vi "Read Slider Props.vi"(8 "error in (no error)":errorcluster, 11 "Slider in":refnum<vi>) -> (0 "error out":errorcluster, 2 "Slider Props":T1, 3 "Slider":refnum<vi>)   [LabVIEW 2020, in "VolatusGUIEditorCore.lvlib"]
uses:
  VolatusGUIEditorCore.lvlib
  Slider Props.ctl
  Fill Style.ctl
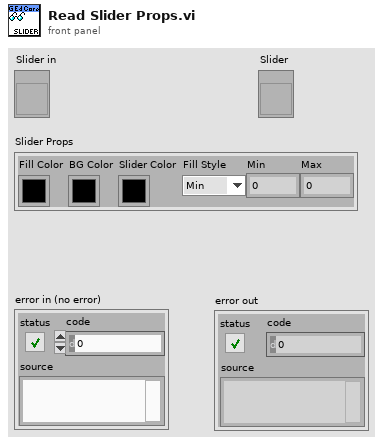
[diagram p1: front panel]
types:
  T1 = typedef "VolatusGUIEditorCore.lvlib/Slider Props.ctl" = cluster{"Fill Color":u32, "BG Color":u32, "Slider Color":u32, "Fill Style":T2, "Min":dbl, "Max":dbl}
  T2 = typedef "VolatusGUIEditorCore.lvlib/Fill Style.ctl" = enum16{"Min", "Max", "None"}
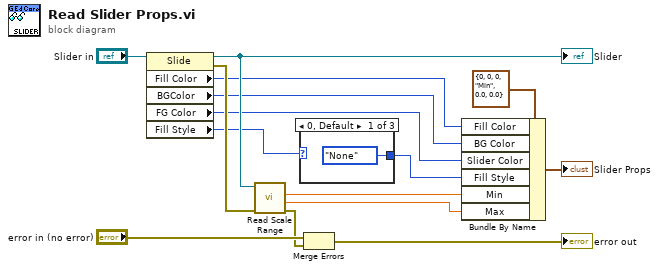
[diagram p0: block diagram]
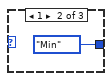
[diagram p2: hidden frame]
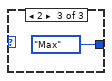
[diagram p3: hidden frame]
diagram:
  n1 = property class="Slide"(reference="Slider in") -> (reference out=w13:refnum<vi>, error out=w15:errorcluster, "Fill Color"=w10:u32, "BGColor"=w9:u32, "FG Color"=w8:u32, "Fill Style"=w5:i32)  [unwired: 1 in]
  "Slider" <- w13
  n2 = call "Read Scale Range.vi"("error in (no error)"=w15, "Ctl Refnum in"=w13) -> ("error out"=w3:errorcluster, "Max"=w6:dbl, "Min"=w7:dbl)  [unwired: 6 in, 1 out]
  n3 = case shown="0, Default" w5 {
    tunnel: [Fill_Style."None" ("Fill Style") Fill_Style."Min" ("Fill Style") Fill_Style."Max" ("Fill Style")] -> w1
    frame 0, Default {
    }
    frame 1 {
    }
    frame 2 {
    }
  }
  n4 = Merge Errors("error in (no error)", w3) -> (→"error out":errorcluster)
  n5 = Bundle By Name(cluster=T1 {"Fill Color"=0, "BG Color"=0, "Slider Color"=0, "Fill Style"=enum."Min", "Min"=0.0, "Max"=0.0} ("Slider Props"), "Fill Color"=w10, "BG Color"=w9, "Slider Color"=w8, "Fill Style"=w1, "Min"=w7, "Max"=w6) -> (→"Slider Props":T1)
